vi "Deserialise content.vi"(8 "error in (no error)":errorcluster, 10 "JSON String to decode":string, 11 "object in":refnum<class "shutdown_reply Message.lvclass">) -> (0 "error out":errorcluster, 3 "object out":refnum<class "shutdown_reply Message.lvclass">)   [LabVIEW 2018, in "ClientMessaging.lvlib" / "shutdown_reply Message.lvclass"]
uses:
  shutdown_reply Message.lvclass
  C:/Users/gavin/Documents/LabVIEW Data/LabVIEW-Bits/Connectivity/Jupyter Client/Base Classes/Reply Message/Reply Message.lvclass
  shutdown_reply Message.lvclass/shutdown_reply Message.ctl
  cf140ef3-bdff-4be1-b5e2-78320a81d22f.vi
  cf140ef3-bdff-4be1-b5e2-78320a81d22f.vi/cba40f93-e8a1-42f9-8302-b6f5020e6cae.vi
  cf140ef3-bdff-4be1-b5e2-78320a81d22f.vi/8e1fc6a5-c839-47be-947f-605362d6cbcd.vi
  cf140ef3-bdff-4be1-b5e2-78320a81d22f.vi/fd355310-4c79-42d4-ad19-5f6a95d9f5f1.vi
  <vilib>/JDP Science/JSONtext/Find Item.vi
  <vilib>/JDP Science/JSONtext/String Subset.vi
  <vilib>/JDP Science/JSONtext/Parsing/Parse Full Path or Item Name.vi
  <vilib>/JDP Science/JSONtext/Offset/Find Item Locations by Path.vi
  <vilib>/JDP Science/JSONtext/JSON text to Variant.vi
  Base Classes/Message Class/Message Class.lvclass
  Base Classes/Reply Message/Reply Message.lvclass
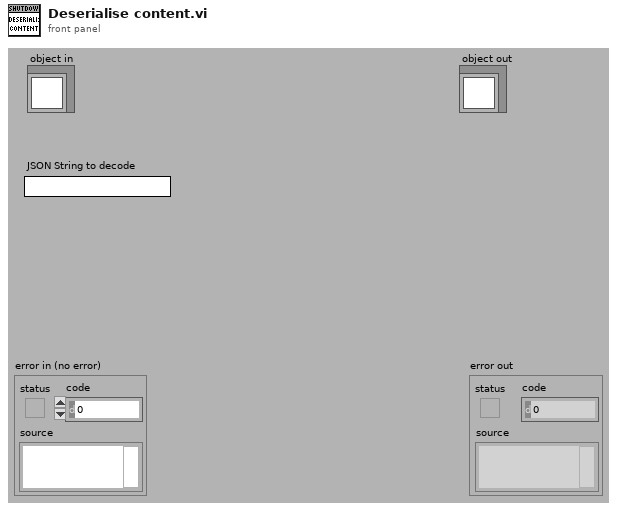
[diagram p1: front panel]
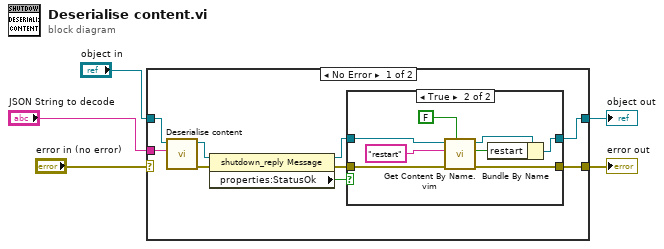
[diagram p0: block diagram]
diagram:
  n1 = case shown="No Error" "error in (no error)" {
    selector: "error in (no error)" -> [_ w26]
    tunnel: [w6 w26] -> w4
    tunnel: [w7 w25] -> w2
    tunnel: "object in" -> [w14 w25]
    tunnel: "JSON String to decode" -> [w12 _]
    frame No Error {
      n2 = call-parent "Deserialise content.vi"("JSON String to decode"=w12, "object in"=w14) -> ("error out"=w11:errorcluster, "object out"=w13:refnum<class "shutdown_reply Message.lvclass">)  [unwired: 8 in]
      n3 = property class="shutdown_reply Message"(reference=w13, error in=w11) -> (reference out=w9:refnum<class "shutdown_reply Message.lvclass">, error out=w8:errorcluster, "properties:StatusOk"=w10:bool)
      n4 = case shown="True" w10 {
        tunnel: w9 -> [w16 w22]
        tunnel: w8 -> [w15 w23]
        tunnel: [w16 w24] -> w7
        tunnel: [w15 w17] -> w6
        frame False {
        }
        frame True {
          n5 = call "Get Content By Name.vim"("Type of content"=FALSE, "error in (no error)"=w23, "Name of Content Item"="restart" ("Element Name"), "Message In"=w22) -> ("error out"=w17:errorcluster, "Data Out"=w19:bool, "Message Out"=w18:refnum<class "shutdown_reply Message.lvclass">)  [unwired: 5 in]
          n6 = Bundle By Name(cluster=w18, "restart"=w19) -> (w24:refnum<class "shutdown_reply Message.lvclass">)
        }
      }
    }
    frame Error {
    }
  }
  "error out" <- w4
  "object out" <- w2
